vi "Create Windows Message Queue.vi"(2 "error in (no error)":errorcluster, 3 "Messeges (none)":u32[](array[numeric]) format="%.0x", 4 "VI Name (Calling VI)":string) -> (0 "error out":errorcluster, 1 "win msg queue":T1)   [LabVIEW 2017, in "Windows messages for Labview (32 and 64).lvlib"]
doc: "Creates a new Windows Message Queue. The queue stores all messages that match any listed in the \"Messages\" input array that are passed to the \"Window Name\" window. The messages can later be retreived from the queue using Wait on Windows Message.vi\n\nParameters:\n\nMessages: The messages that should be queued. For a list of standard windows messages, see the readme file or winuser.h. Default will detect no messages.\n\nWindow Name: Specifies which VI's front panel to monitor. Defaults to the calling VI.\n\nwin msg queue: The new win msg queue refnum.\n\nErrors:\nReturns 6750 if the queue cannot be created."
uses:
  Windows messages for Labview (32 and 64).lvlib
  Win Msg Queue RefNum.ctl
  Windows Messages for LabVIEW_64.dll
  Windows Messages for LabVIEW_32.dll
panel:
  in  "dummy win msg queue":T1
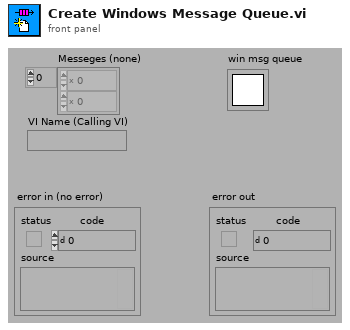
[diagram p1: front panel]
types:
  T1 = typedef "Windows messages for Labview (32 and 64).lvlib/Win Msg Queue RefNum.ctl" = refnum<k1>
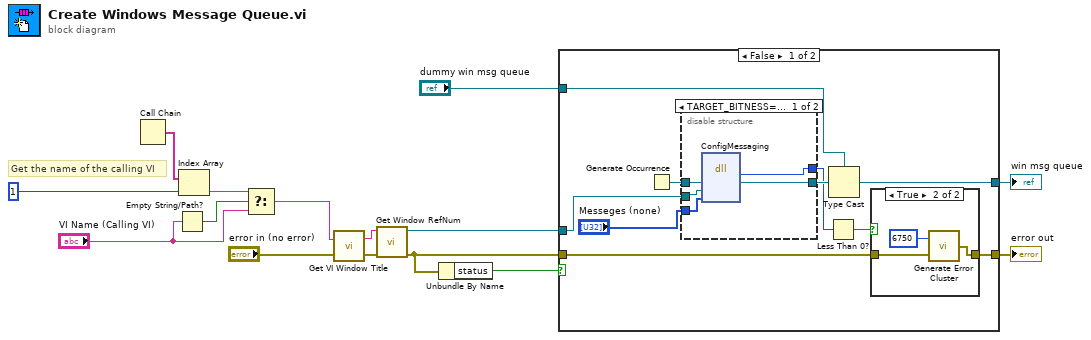
[diagram p0: block diagram]
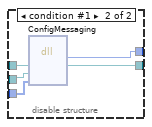
[diagram p2: hidden frame]
diagram:
  # "Get the name of the calling VI"
  n1 = Call Chain() -> (call chain=w15:string[])
  n2 = Empty String/Path?(string/path="VI Name (Calling VI)") -> (empty?=w13:bool)
  n3 = Index Array(array=w15, index=1 ("Index")) -> (element=w12:string)
  n4 = Select(t=w12, s=w13, f="VI Name (Calling VI)") -> (s? t:f=w6:string)
  n5 = call "Get VI Window Title.vi"("error in (no error)"="error in (no error)", "VI Name"=w6) -> ("error out"=w3:errorcluster, "Window Title"=w4:string)
  n6 = call "Get Window RefNum.vi"("error in (no error)"=w3, "window name (\"\")"=w4) -> ("error out"=w2:errorcluster, "Window Refnum"=w1:T1)  [unwired: 6 in]
  n7 = Unbundle By Name(w2) -> ("status"=w10:bool)
  n8 = case shown="False" w10 {
    tunnel: w1 -> [w20 _]
    tunnel: w2 -> [w24 w41]
    tunnel: [w23 w41] -> w9
    tunnel: [w21 w40] -> w7
    tunnel: "dummy win msg queue" -> [w22 w40]
    frame False {
      n9 = Generate Occurrence() -> (w19:refnum<k4>)
      n10 = disable-structure shown="TARGET_BITNESS==64, Default" {
        disable-tunnel: [w28 w32] -> w17
        disable-tunnel: [w27 w31] -> w16
        disable-tunnel: w20 -> [w30 w34]
        disable-tunnel: w19 -> [w29 w35]
        disable-tunnel: "Messeges (none)" -> [w26 w33]
        frame condition #0 (active) {
          n11 = dll-call lib="M:/_dev/progs/LabVIEW/_lib/Windows Messages for Labview/llb/Windows Messages for LabVIEW_64.dll" fn="ConfigMessaging"("occurrence"=w29, "hWnd"=w30, "arg3"=w26) -> ("return type"=w27:i32, "occurrence"=w28:refnum<k4>)  [unwired: 5 in, 2 out]
        }
        frame condition #1 {
          n12 = dll-call lib="D:/labview_d/temp/Windows Messaging/Windows Messages for Labview/llb/Windows Messages for LabVIEW_32.dll" fn="ConfigMessaging"("occurrence"=w35, "hWnd"=w34, "arg3"=w33) -> ("return type"=w31:i32, "occurrence"=w32:refnum<k4>)  [unwired: 5 in, 2 out]
        }
      }
      n13 = Less Than 0?(x=w16) -> (x < 0?=w25:bool)
      n14 = Type Cast(type=w22, x=w17) -> (*(type *) &x=w21:T1)
      n15 = case shown="True" w25 {
        tunnel: w24 -> [w36 w38]
        tunnel: [w36 w39] -> w23
        frame False {
        }
        frame True {
          n16 = call "Generate Error Cluster.vi"("error in (no error)"=w38, "Error Code"=6750) -> ("error out"=w39:errorcluster)
        }
      }
    }
    frame True {
    }
  }
  "win msg queue" <- w7
  "error out" <- w9
